vi "Choose Manual Shot Type.vi"(8 "1":bool, 9 "2":bool, 10 "3":bool, 11 "4":bool) -> (2 "Manual Shot?":bool, 3 "Manual Shot Distance":dbl)   [LabVIEW 2025]
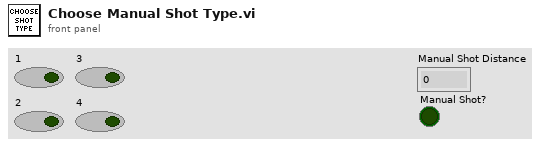
[diagram p1: front panel]
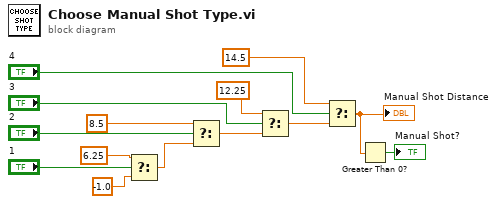
[diagram p0: block diagram]
diagram:
  n1 = Select(t=6.25, s="1", f=-1.0) -> (s? t:f=w12:dbl)
  n2 = Select(t=8.5, s="2", f=w12) -> (s? t:f=w10:dbl)
  n3 = Select(t=12.25, s="3", f=w10) -> (s? t:f=w8:dbl)
  n4 = Select(t=14.5, s="4", f=w8) -> (s? t:f=w2:dbl)
  "Manual Shot Distance" <- w2
  n5 = Greater Than 0?(x=w2) -> (x > 0?=→"Manual Shot?":bool)
